vi "Main.vi"() -> ()   [LabVIEW 2013]
uses:
  <vilib>/myRIO/Instrument Drivers/Onboard IO/DIO/vis/Smart Open.vi
  <vilib>/myRIO/Instrument Drivers/Onboard IO/DIO/vis/Read.vi
  <vilib>/myRIO/Instrument Drivers/Onboard IO/DIO/vis/Write.vi
  <vilib>/myRIO/Common/Instrument Driver Framework/myRIO v1.0/UART/vis/myRIO v1.0 Close UART.vi
  <vilib>/myRIO/Instrument Drivers/Onboard IO/DIO/vis/Open.vi
  <vilib>/myRIO/Common/Instrument Driver Framework/myRIO v1.0/DIO/vis/myRIO v1.1 Open DIO.vi
  <vilib>/myRIO/Common/Instrument Driver Framework/Utilities/vis/Validate Channels.vi
  <vilib>/myRIO/Common/Instrument Driver Framework/myRIO v1.0/DIO/vis/myRIO v1.0 Reserve DIO.vi
  <vilib>/myRIO/Common/Instrument Driver Framework/myRIO v1.0/Resource Manager/vis/myRIO v1.0 Reserve Channel List.vi
  <vilib>/myRIO/Common/Instrument Driver Framework/myRIO v1.0/DIO/vis/myRIO v1.0 Build MUX Configuration DIO.vi
  <vilib>/myRIO/Common/Instrument Driver Framework/myRIO v1.0/Resource Manager/vis/myRIO v1.0 Reserve Channel.vi
  <vilib>/myRIO/Common/Instrument Driver Framework/myRIO v1.0/Resource Manager/vis/myRIO v1.0 Unreserve Channel.vi
  <vilib>/myRIO/Common/Instrument Driver Framework/myRIO v1.0/Resource Manager/vis/myRIO v1.0 Create Configuration List.vi
  <vilib>/myRIO/Common/Instrument Driver Framework/myRIO v1.0/Resource Manager/vis/myRIO v1.0 Build Mutex Name.vi
  <vilib>/Instr/_visa.llb/VISA Configure Serial Port (Instr).vi
  <vilib>/myRIO/Common/Instrument Driver Framework/myRIO v1.0/myRIO v1.1 Open.vi
  <vilib>/Utility/VariantDataType/GetNumericInfo.vi
  <vilib>/Utility/error.llb/Error Cluster From Error Code.vi
  <vilib>/myRIO/Common/Instrument Driver Framework/Utilities/vis/IO Manager.vi
  <vilib>/myRIO/Common/Instrument Driver Framework/Utilities/vis/Configuration Manager.vi
  <vilib>/myRIO/Common/Instrument Driver Framework/myRIO v1.0/Resource Manager/vis/myRIO v1.0 Configure IO.vi
  <vilib>/myRIO/Common/Instrument Driver Framework/myRIO v1.0/myRIO v1.0 Close.vi
  <vilib>/myRIO/Common/Instrument Driver Framework/myRIO v1.0/DIO/vis/myRIO v1.0 Write DIO.vi
  <vilib>/myRIO/Common/Instrument Driver Framework/myRIO v1.0/DIO/vis/myRIO v1.0 Read DIO.vi
  <vilib>/myRIO/Common/Instrument Driver Framework/Utilities/vis/FPGA Ref Manager.vi
  <vilib>/myRIO/Common/Instrument Driver Framework/myRIO v1.0/myRIO v1.0 Reset FPGA.vi
  <vilib>/myRIO/Instrument Drivers/Utilities/Utilities.lvlib
panel:
  in  "enable echo":bool
  out "ASCII hex code":u8 format="%02x"
  in  "CTS":bool
  out "incoming\ncharacter":string
  out "RTS":bool
  in  "RESET":bool
  out "STATUS":bool
  in  "[ESC]":bool
  # "Bluetooth demo"
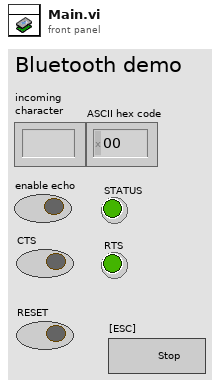
[diagram p1: front panel]
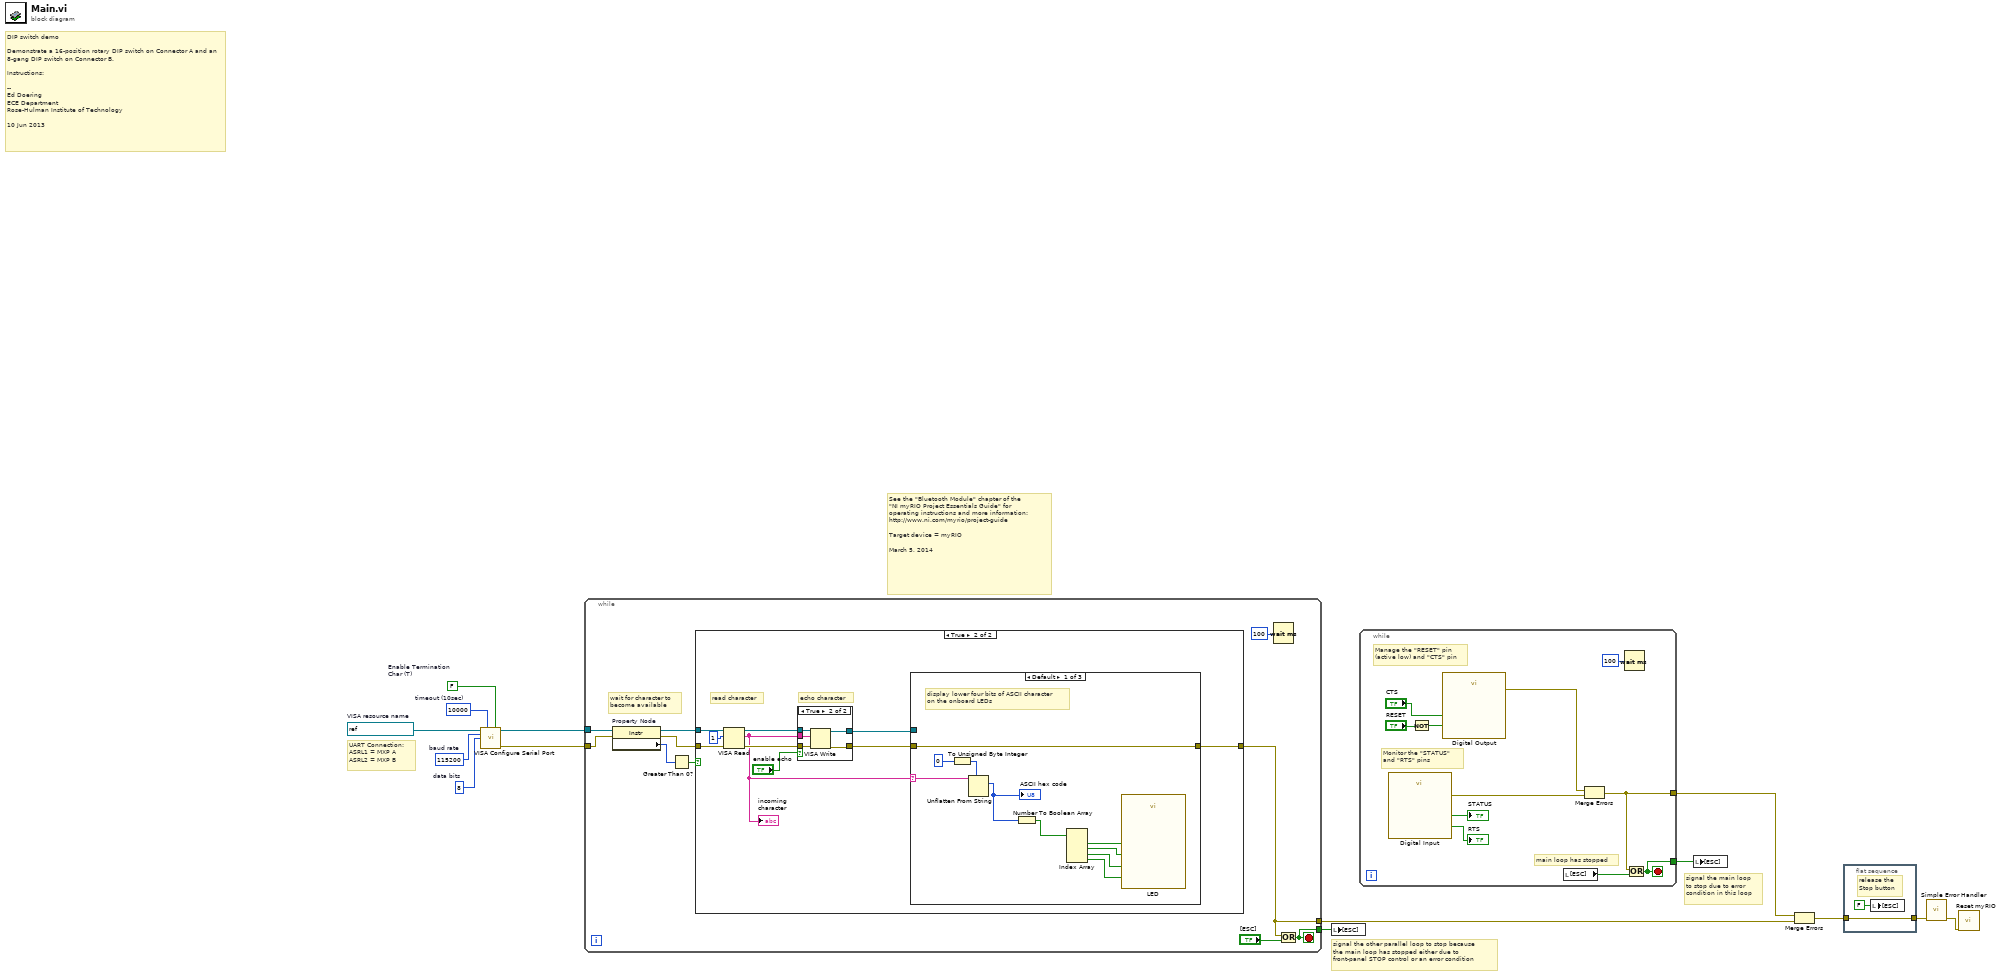
[diagram p0: block diagram]
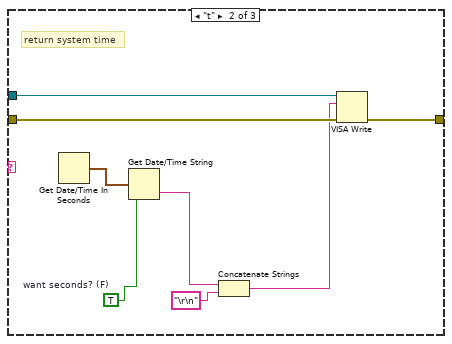
[diagram p4: hidden frame]
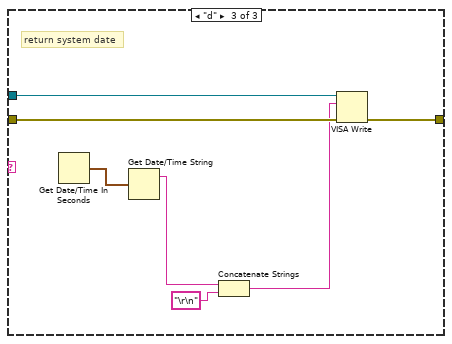
[diagram p5: hidden frame]
diagram:
  w1 = u32 10000  # timeout (10sec)
  w4 = FALSE  # Enable Termination Char (T)
  w10 = u16 8  # data bits
  w11 = u32 115200  # baud rate
  w13 = refnum<visa-resource-name> "ASRL2::INSTR"  # VISA resource name
  # "See the \"Bluetooth Module\" chapter of the\n\"NI myRIO Project Essentials Guide\" for\noperating instructions and more information: \nhttp://www.ni.com/myrio/project-guide\n\nTarget device = myRIO\n\nMarch 5, 2014"
  # "signal the main loop\nto stop due to error\ncondition in this loop"
  # "signal the other parallel loop to stop because\nthe main loop has stopped either due to\nfront-panel STOP control or an error condition"
  # "UART Connection:\nASRL1 = MXP A \nASRL2 = MXP B"
  # "DIP switch demo\n\nDemonstrate a 16-position rotary DIP switch on Connector A and an 8-gang DIP switch on Connector B.\n\nInstructions:\n\n-- \nEd Doering\nECE Department\nRose-Hulman Institute of Technology\n\n10 Jun 2013"
  n1 = call-poly "VISA Configure Serial Port"("VISA resource name"=w13, "timeout (10sec)"=w1, "Enable Termination\nChar (T)"=w4, "baud rate (9600)"=w11, "data bits (8)"=w10) -> ("VISA resource name out"=w12:refnum<visa-resource-name>, "error out"=w7:errorcluster)  [unwired: 9 in]
  n2 = while {
    tunnel: [w22] -> w9
    tunnel: w12 -> [w20]
    tunnel: w7 -> [w19]
    tunnel: [w21] -> w6
    stop <- w21 stop-if-true
    # "wait for character to\nbecome available"
    n3 = property on="Property Node" class="Instr"(reference=w20, error in=w19) -> (reference out=w15:refnum<visa-resource-name>, error out=w18:errorcluster, "Serial Settings:Number of Bytes at Serial Port"=w17:u32)
    n4 = Greater Than 0?(x=w17) -> (x > 0?=w16:bool)
    n5 = case shown="True" w16 {
      tunnel: [w25 w35] -> w22
      tunnel: w18 -> [w25 w33]
      tunnel: w15 -> [_ w32]
      frame False {
      }
      frame True {
        # "echo character"
        # "read character"
        n6 = VISA Read(VISA resource name=w32, byte count=u32 1, error in (no error)=w33) -> (VISA resource name out=w30:refnum<visa-resource-name>, read buffer=w26:string, error out=w31:errorcluster)  [unwired: 1 out]
        "incoming\ncharacter" <- w26
        n7 = case shown="True" "enable echo" {
          tunnel: w31 -> [w36 w42]
          tunnel: w26 -> [_ w41]
          tunnel: w30 -> [w37 w40]
          tunnel: [w37 w39] -> w29
          tunnel: [w36 w38] -> w27
          frame False {
          }
          frame True {
            n8 = VISA Write(VISA resource name=w40, write buffer=w41, error in (no error)=w42) -> (VISA resource name out=w39:refnum<visa-resource-name>, error out=w38:errorcluster)  [unwired: 1 out]
          }
        }
        n9 = case shown="Default" w26 {
          selector: w26 -> [w50 _ _]
          tunnel: w27 -> [w52 w57 w65]
          tunnel: [w52 w56 w64] -> w35
          tunnel: w29 -> [_ w58 w66]
          frame Default {
            # "display lower four bits of ASCII character\non the onboard LEDs"
            n10 = To Unsigned Byte Integer(number=u8 0) -> (unsigned 8bit integer=w49:u8)
            n11 = Unflatten From String(type=w49, binary string=w50) -> (value=w43:u8)  [unwired: 3 in, 2 out]
            "ASCII hex code" <- w43
            n12 = Number To Boolean Array(number=w43) -> (Boolean array=w48:bool[])
            n13 = Index Array "Index Array"(array=w48) -> (element #1=w47:bool, element #2=w46:bool, element #3=w45:bool, element #4=w44:bool)  [unwired: 4 in]
            n14 = call "LED"("LED0"=w47, "LED1"=w46, "LED2"=w45, "LED3"=w44) -> ()  [unwired: 23 in, 1 out]
          }
          frame "t" {
            w60 = TRUE  # want seconds? (F)
            # "return system time"
            n15 = Get Date/Time In Seconds() -> (seconds since 1Jan1904=w59:timestamp)
            n16 = Get Date/Time String(seconds (now)=w59, want seconds? (F)=w60) -> (time string=w55:string)  [unwired: 1 in, 1 out]
            n17 = Concatenate Strings "Concatenate Strings"(w55, "\r\n" ("string")) -> (w53:string)
            n18 = VISA Write(VISA resource name=w58, write buffer=w53, error in (no error)=w57) -> (error out=w56:errorcluster)  [unwired: 2 out]
          }
          frame "d" {
            # "return system date"
            n19 = Get Date/Time In Seconds() -> (seconds since 1Jan1904=w67:timestamp)
            n20 = Get Date/Time String(seconds (now)=w67) -> (date string=w61:string)  [unwired: 2 in, 1 out]
            n21 = Concatenate Strings "Concatenate Strings"(w61, "\r\n" ("string")) -> (w62:string)
            n22 = VISA Write(VISA resource name=w66, write buffer=w62, error in (no error)=w65) -> (error out=w64:errorcluster)  [unwired: 2 out]
          }
        }
      }
    }
    n23 = Wait (ms)(milliseconds to wait=u32 100) -> ()  [unwired: 1 out]
    n24 = Or(x=w22, y="[ESC]") -> (x .or. y?=w21:bool)
  }
  n25 = local write "[ESC]"(w6) -> ()
  n26 = while {
    tunnel: [w73] -> w8
    tunnel: [w75] -> w5
    stop <- w75 stop-if-true
    # "Manage the \"RESET\" pin\n(active low) and \"CTS\" pin"
    # "main loop has stopped"
    # "Monitor the \"STATUS\"\nand \"RTS\" pins"
    n27 = call "Digital Input"() -> ("B/DIO0 (Pin 11)"=→"STATUS":bool, "B/DIO1 (Pin 13)"=→"RTS":bool, "error out"=w70:errorcluster)  [unwired: 25 in]
    n28 = Not(x="RESET") -> (.not. x?=w69:bool)
    n29 = call "Digital Output"("B/DIO2 (Pin 15)"="CTS", "B/DIO3 (Pin 17)"=w69) -> ("error out"=w74:errorcluster)  [unwired: 25 in]
    n30 = local read "[ESC]"() -> (w76:bool)
    n31 = Merge Errors "Merge Errors"(w74, w70) -> (w73:errorcluster)
    n32 = Wait (ms)(milliseconds to wait=u32 100) -> ()  [unwired: 1 out]
    n33 = Or(x=w73, y=w76) -> (x .or. y?=w75:bool)
  }
  n34 = local write "[ESC]"(w5) -> ()
  n35 = Merge Errors "Merge Errors"(w8, w9) -> (w3:errorcluster)
  n36 = flat-sequence {
    tunnel: w3 -> [w79]
    tunnel: [w79] -> w2
    frame #0 {
      # "release the\nStop button"
      n37 = local write "[ESC]"(FALSE ("[ESC]")) -> ()
    }
  }
  n38 = call <vilib>:"Simple Error Handler.vi"("error in (no error)"=w2) -> ("error out"=w14:errorcluster)  [unwired: 4 in, 4 out]
  n39 = call <vilib>:"Reset myRIO.vi"("error in (no error)"=w14) -> ()  [unwired: 10 in, 1 out]
